vi "Get Library Path.vi"(8 "error in (no error)":errorcluster) -> (0 "error out":errorcluster, 3 "Path":path)   [LabVIEW 2017]
uses:
  Source/Classes/Pointer/Pointer.lvclass
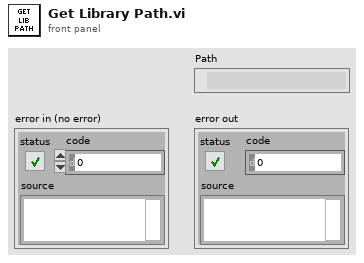
[diagram p1: front panel]
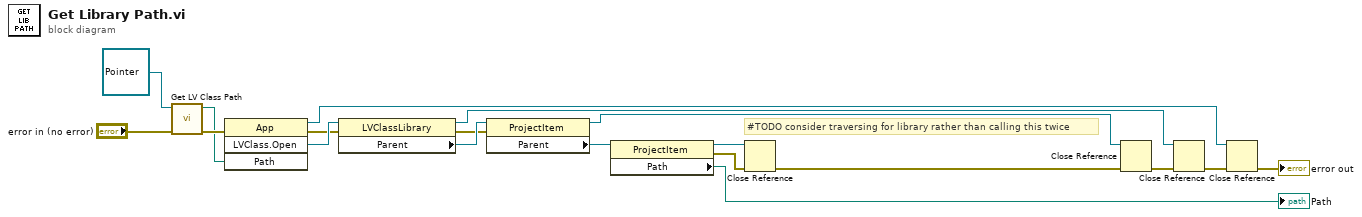
[diagram p0: block diagram]
diagram:
  # "#TODO consider traversing for library rather than calling this twice"
  n1 = call <vilib>:"Get LV Class Path.vi"("error in (no error)"="error in (no error)", "object"=refnum<class "Pointer.lvclass"> refnum ("Memory Manager.lvlib:Pointer")) -> ("error out"=w19:errorcluster, "class path"=w17:path)  [unwired: 8 in]
  n2 = invoke class="App" method="LVClass.Open"(error in=w19, "Path"=w17) -> (reference out=w6:refnum<vi>, error out=w2:errorcluster, "LVClass.Open"=w12:refnum<vi>)  [unwired: 2 in, 1 out]
  n3 = property class="LVClassLibrary"(reference=w12, error in=w2) -> (reference out=w7:refnum<vi>, error out=w1:errorcluster, "Parent"=w15:refnum<vi>)
  n4 = property class="ProjectItem"(reference=w15, error in=w1) -> (reference out=w8:refnum<vi>, "Parent"=w14:refnum<vi>)  [unwired: 1 out]
  n5 = property class="ProjectItem"(reference=w14) -> (reference out=w10:refnum<vi>, error out=w11:errorcluster, "Path"=→"Path":path)  [unwired: 1 in]
  n6 = Close Reference(reference=w10, error in (no error)=w11) -> (error out=w9:errorcluster)
  n7 = Close Reference(reference=w8, error in (no error)=w9) -> (error out=w5:errorcluster)
  n8 = Close Reference(reference=w7, error in (no error)=w5) -> (error out=w4:errorcluster)
  n9 = Close Reference(reference=w6, error in (no error)=w4) -> (error out=→"error out":errorcluster)
